vi "Sensitivity.vi"(9 "Power (z)":dbl min=0.0 step=0.1, 10 "Sensitivity (a)":dbl step=0.1, 11 "Input":dbl(slide) scale=-1.0..1.0) -> (3 "Output":dbl(slide) scale=-1.0..1.0)   [LabVIEW 2016]
panel:
  out "XY Graph":cluster{dbl[], dbl[]}(graph)
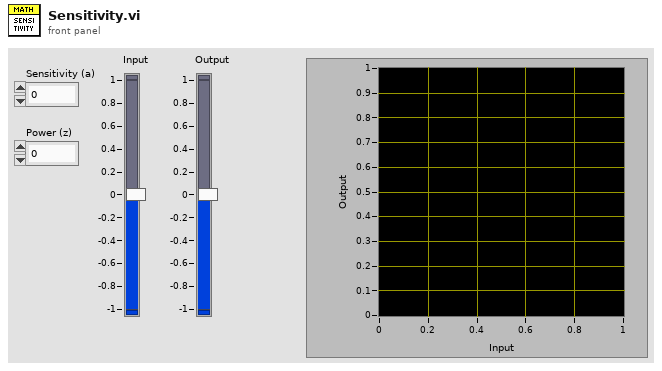
[diagram p1: front panel]
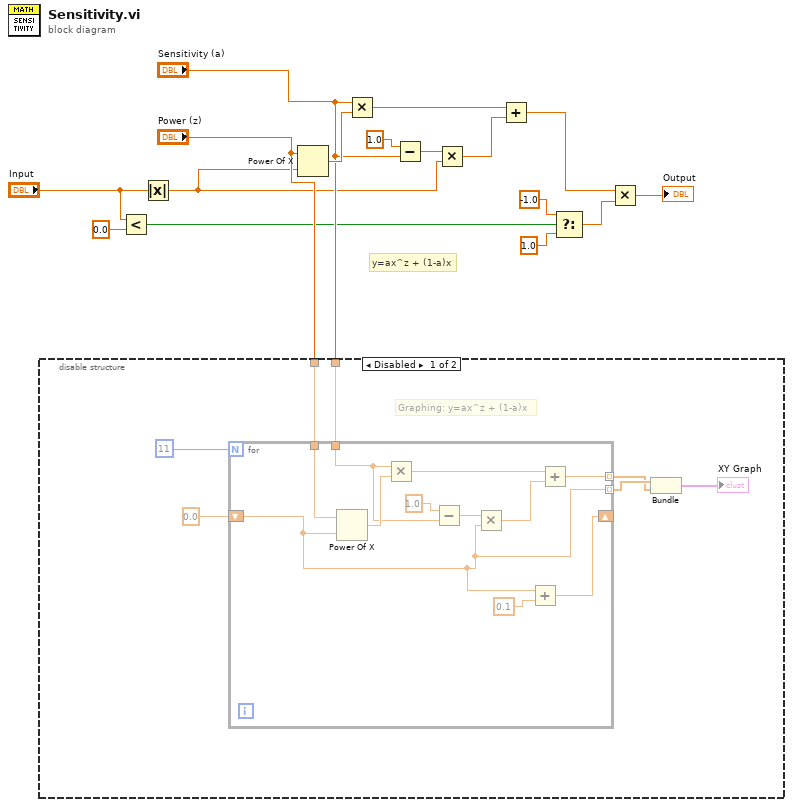
[diagram p0: block diagram]
diagram:
  # "y=ax^z + (1-a)x"
  n1 = disable-structure shown="Disabled" {
    disable-tunnel: "Sensitivity (a)" -> [w23 _]
    disable-tunnel: "Power (z)" -> [w22 _]
    frame Disabled {
      # "Graphing: y=ax^z + (1-a)x"
      n2 = for {
        N: 11 -> [_]
        shift-right: [w26] -> _
        shift-left: 0.0 -> [w24]
        tunnel: w23 -> [w29]
        tunnel: w22 -> [w28]
        tunnel: [w25] -> w18 mode=indexing
        tunnel: [w24] -> w19 mode=indexing
        n3 = Power Of X(1:w24, 2:w28) -> (0:w34:dbl)
        n4 = Multiply(x=w29, y=w34) -> (x*y=w33:dbl)
        n5 = Subtract(x=1.0, y=w29) -> (x-y=w31:dbl)
        n6 = Multiply(x=w31, y=w24) -> (x*y=w30:dbl)
        n7 = Add(x=w24, y=0.1) -> (x+y=w26:dbl)
        n8 = Add(x=w33, y=w30) -> (x+y=w25:dbl)
      }
      n9 = Bundle(w19, w18) -> (→"XY Graph":cluster{dbl[], dbl[]})  [unwired: 1 in]
    }
    frame Enabled {
    }
  }
  n10 = Less?(x="Input", y=0.0) -> (x < y?=w3:bool)
  n11 = Absolute Value(x="Input") -> (abs(x)=w1:dbl)
  n12 = Power Of X(1:w1, 2:"Power (z)") -> (0:w16:dbl)
  n13 = Multiply(x="Sensitivity (a)", y=w16) -> (x*y=w15:dbl)
  n14 = Subtract(x=1.0, y="Sensitivity (a)") -> (x-y=w13:dbl)
  n15 = Multiply(x=w13, y=w1) -> (x*y=w12:dbl)
  n16 = Add(x=w15, y=w12) -> (x+y=w8:dbl)
  n17 = Select(t=-1.0, s=w3, f=1.0) -> (s? t:f=w6:dbl)
  n18 = Multiply(x=w8, y=w6) -> (x*y=→"Output":dbl)
